vi "Tree.vi"(8 "error in (no error)":errorcluster, 11 "Instrument.Oxford1820":refnum<class "Instrument.OxfordVRM.lvclass">) -> (0 "error out":errorcluster, 3 "Instrument.Oxford1820 out":refnum<class "Instrument.OxfordVRM.lvclass">)   [LabVIEW 2016, in "Instrument.OxfordVRM.lvclass"]
uses:
  Instrument.OxfordVRM.lvclass
  Instrument.Oxford1820 UI/Instrument.OxfordVRM UI.lvclass
  Typedefs/Instrument.Oxford1820.Commands-enum.ctl
  <userlib>/LevyLab/Levylab Instruments/SMOs/Instrument/Instrument.lvclass
  <userlib>/LevyLab/Levylab Instruments/SMOs/RemoteControl/RemoteControl.lvclass
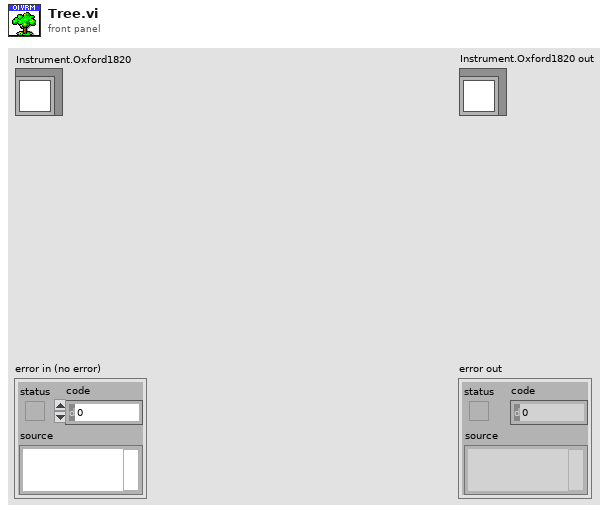
[diagram p1: front panel]
types:
  T1 = typedef "Instrument.OxfordVRM.lvclass/Instrument.Oxford1820.Commands-enum.ctl" = enum16{"setAction", "setTarget", "setSwitchHeat", "setLambda", "setFillMode", "setNeedleValve", "setMagnetField", "getStatus", "getTarget", "getSwitchHeat", "getPSUField", "newcommand", "getMagnetField"}
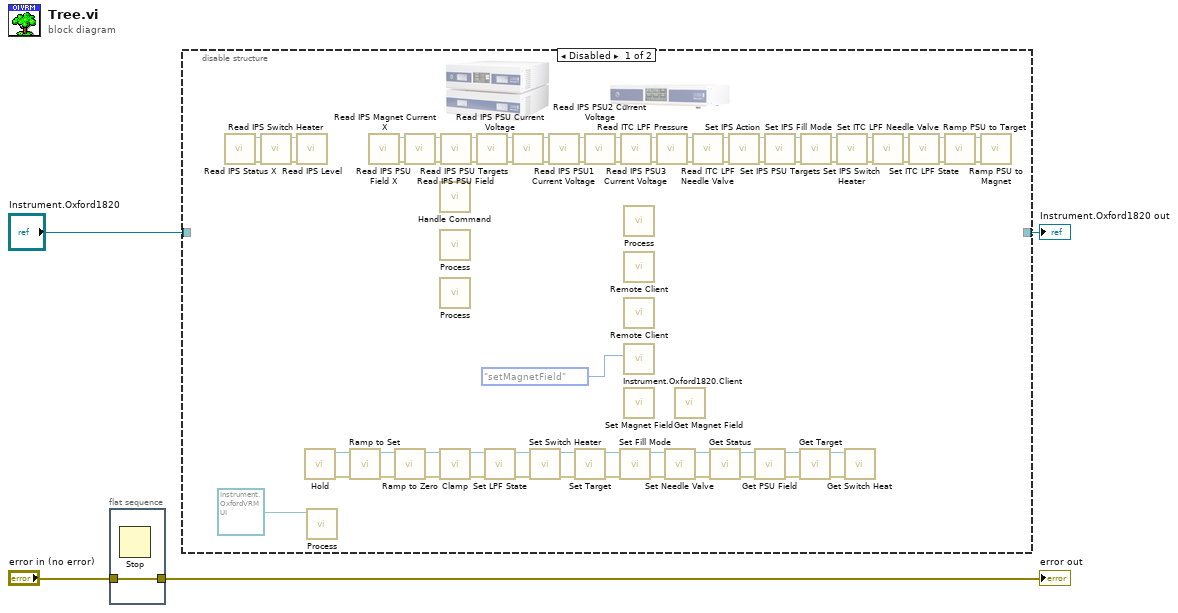
[diagram p0: block diagram]
diagram:
  n1 = flat-sequence {
    tunnel: "error in (no error)" -> [w5]
    tunnel: [w5] -> w4
    frame #0 {
      n2 = Stop() -> ()  [unwired: 1 in]
    }
  }
  n3 = disable-structure shown="Disabled" {
    disable-tunnel: [_ w70] -> w3
    disable-tunnel: "Instrument.Oxford1820" -> [_ w70]
    frame Disabled {
      n4 = call "Read IPS Status X.vi"() -> ("error out"=w67:errorcluster, "Instrument.OxfordVRM out"=w68:refnum<class "Instrument.OxfordVRM.lvclass">)  [unwired: 9 in, 1 out]
      n5 = call "Read IPS Switch Heater.vi"("error in (no error)"=w67, "Instrument.Oxford1820 in"=w68) -> ("error out"=w65:errorcluster, "Instrument.Oxford1820 out"=w66:refnum<class "Instrument.OxfordVRM.lvclass">)  [unwired: 6 in, 2 out]
      n6 = call "Read IPS Level.vi"("error in (no error)"=w65, "Instrument.Oxford1820 in"=w66) -> ()  [unwired: 6 in, 4 out]
      n7 = call "Hold.vi"() -> ("error out"=w33:errorcluster, "Instrument.1820 in"=w34:refnum<class "Instrument.OxfordVRM.lvclass">)  [unwired: 9 in, 1 out]
      n8 = call-dynamic "Process.vi"("Oxford1820 UI in"=refnum<class "Instrument.OxfordVRM UI.lvclass"> refnum ("Instrument.Oxford1820 UI.lvclass")) -> ()  [unwired: 9 in, 2 out]
      n9 = call "Ramp to Set.vi"("error in (no error)"=w33, "Instrument.1820 in"=w34) -> ("error out"=w31:errorcluster, "Instrument.1820 in"=w32:refnum<class "Instrument.OxfordVRM.lvclass">)  [unwired: 7 in, 1 out]
      n10 = call "Read IPS PSU Field X.vi"() -> ("error out"=w63:errorcluster, "Instrument.OxfordVRM out"=w64:refnum<class "Instrument.OxfordVRM.lvclass">)  [unwired: 9 in, 1 out]
      n11 = call "Ramp to Zero.vi"("error in (no error)"=w31, "Instrument.1820 in"=w32) -> ("error out"=w29:errorcluster, "Instrument.1820 in"=w30:refnum<class "Instrument.OxfordVRM.lvclass">)  [unwired: 7 in, 1 out]
      n12 = call "Read IPS Magnet Current X.vi"("error in (no error)"=w63, "Instrument.OxfordVRM in"=w64) -> ("error out"=w61:errorcluster, "Instrument.OxfordVRM out"=w62:refnum<class "Instrument.OxfordVRM.lvclass">)  [unwired: 7 in, 1 out]
      n13 = call-dynamic "Handle Command.vi"() -> ()  [unwired: 8 in, 4 out]
      n14 = call-dynamic "Process.vi"() -> ()  [unwired: 10 in, 2 out]
      n15 = call-dynamic "Process.vi"() -> ()  [unwired: 10 in, 2 out]
      n16 = call "Clamp.vi"("error in (no error)"=w29, "Instrument.1820 in"=w30) -> ("error out"=w27:errorcluster, "Instrument.1820 in"=w28:refnum<class "Instrument.OxfordVRM.lvclass">)  [unwired: 7 in, 1 out]
      n17 = call "Read IPS PSU Field.vi"("error in (no error)"=w61, "Instrument.OxfordVRM in"=w62) -> ("error out"=w59:errorcluster, "Instrument.OxfordVRM out"=w60:refnum<class "Instrument.OxfordVRM.lvclass">)  [unwired: 7 in, 1 out]
      n18 = call "Read IPS PSU Targets.vi"("error in (no error)"=w59, "Instrument.OxfordVRM in"=w60) -> ("error out"=w57:errorcluster, "Instrument.OxfordVRM out"=w58:refnum<class "Instrument.OxfordVRM.lvclass">)  [unwired: 6 in, 2 out]
      n19 = call "Set LPF State.vi"("error in (no error)"=w27, "Instrument.1820 in"=w28) -> ("error out"=w25:errorcluster, "Instrument.1820 in"=w26:refnum<class "Instrument.OxfordVRM.lvclass">)  [unwired: 7 in, 1 out]
      n20 = call "Read IPS PSU Current Voltage.vi"("error in (no error)"=w57, "Instrument.OxfordVRM in"=w58) -> ("error out"=w55:errorcluster, "Instrument.OxfordVRM out"=w56:refnum<class "Instrument.OxfordVRM.lvclass">)  [unwired: 6 in, 2 out]
      n21 = call "Set Switch Heater.vi"("error in (no error)"=w25, "Instrument.1820 in"=w26) -> ("error out"=w23:errorcluster, "Instrument.1820 in"=w24:refnum<class "Instrument.OxfordVRM.lvclass">)  [unwired: 7 in, 1 out]
      n22 = call "Read IPS PSU1 Current Voltage.vi"("error in (no error)"=w55, "Instrument.OxfordVRM in"=w56) -> ("error out"=w53:errorcluster, "Instrument.OxfordVRM out"=w54:refnum<class "Instrument.OxfordVRM.lvclass">)  [unwired: 6 in, 2 out]
      n23 = call "Set Target.vi"("error in (no error)"=w23, "Instrument.1820 in"=w24) -> ("error out"=w21:errorcluster, "Instrument.1820 in"=w22:refnum<class "Instrument.OxfordVRM.lvclass">)  [unwired: 7 in, 1 out]
      n24 = call "Read IPS PSU2 Current Voltage.vi"("error in (no error)"=w53, "Instrument.OxfordVRM in"=w54) -> ("error out"=w51:errorcluster, "Instrument.OxfordVRM out"=w52:refnum<class "Instrument.OxfordVRM.lvclass">)  [unwired: 6 in, 2 out]
      n25 = call "Set Fill Mode.vi"("error in (no error)"=w21, "Instrument.1820 in"=w22) -> ("error out"=w8:errorcluster, "Instrument.1820 in"=w9:refnum<class "Instrument.OxfordVRM.lvclass">)  [unwired: 7 in, 1 out]
      n26 = call "Read IPS PSU3 Current Voltage.vi"("error in (no error)"=w51, "Instrument.OxfordVRM in"=w52) -> ("error out"=w49:errorcluster, "Instrument.OxfordVRM out"=w50:refnum<class "Instrument.OxfordVRM.lvclass">)  [unwired: 6 in, 2 out]
      n27 = call-dynamic "Process.vi"() -> ()  [unwired: 10 in, 2 out]
      n28 = call <userlib>:"Remote Client.vi"() -> ()  [unwired: 8 in, 4 out]
      n29 = call <userlib>:"Remote Client.vi"() -> ()  [unwired: 8 in, 4 out]
      n30 = call "Instrument.Oxford1820.Client.vi"("Commands"=Instrument.Oxford1820.Commands-enum."setMagnetField") -> ()  [unwired: 8 in, 3 out]
      n31 = call-dynamic "Set Magnet Field.vi"() -> ()  [unwired: 10 in, 2 out]
      n32 = call "Read ITC LPF Pressure.vi"("error in (no error)"=w49, "Instrument.Oxford1820 in"=w50) -> ("error out"=w47:errorcluster, "Instrument.Oxford1820 out"=w48:refnum<class "Instrument.OxfordVRM.lvclass">)  [unwired: 7 in, 1 out]
      n33 = call "Set Needle Valve.vi"("error in (no error)"=w8, "Instrument.1820 in"=w9) -> ("error out"=w6:errorcluster, "Instrument.1820 in"=w7:refnum<class "Instrument.OxfordVRM.lvclass">)  [unwired: 7 in, 1 out]
      n34 = call-dynamic "Get Magnet Field.vi"() -> ()  [unwired: 7 in, 5 out]
      n35 = call "Read ITC LPF Needle Valve.vi"("error in (no error)"=w47, "Instrument.Oxford1820 in"=w48) -> ("error out"=w45:errorcluster, "Instrument.Oxford1820 out"=w46:refnum<class "Instrument.OxfordVRM.lvclass">)  [unwired: 7 in, 1 out]
      n36 = call "Get Status.vi"("error in (no error)"=w6, "Instrument.1820 in"=w7) -> ("error out"=w19:errorcluster, "Instrument.1820 in"=w20:refnum<class "Instrument.OxfordVRM.lvclass">)  [unwired: 6 in, 2 out]
      n37 = call "Set IPS Action.vi"("error in (no error)"=w45, "Instrument.OxfordVRM in"=w46) -> ("error out"=w43:errorcluster, "Instrument.OxfordVRM out"=w44:refnum<class "Instrument.OxfordVRM.lvclass">)  [unwired: 7 in, 1 out]
      n38 = call "Get PSU Field.vi"("error in (no error)"=w19, "Instrument.1820 in"=w20) -> ("error out"=w17:errorcluster, "Instrument.1820 in"=w18:refnum<class "Instrument.OxfordVRM.lvclass">)  [unwired: 7 in, 1 out]
      n39 = call "Set IPS PSU Targets.vi"("error in (no error)"=w43, "Instrument.OxfordVRM in"=w44) -> ("error out"=w41:errorcluster, "Instrument.OxfordVRM out"=w42:refnum<class "Instrument.OxfordVRM.lvclass">)  [unwired: 7 in, 1 out]
      n40 = call "Get Target.vi"("error in (no error)"=w17, "Instrument.1820 in"=w18) -> ("error out"=w15:errorcluster, "Instrument.1820 in"=w16:refnum<class "Instrument.OxfordVRM.lvclass">)  [unwired: 6 in, 2 out]
      n41 = call "Set IPS Fill Mode.vi"("error in (no error)"=w41, "Instrument.Oxford1820 in"=w42) -> ("error out"=w39:errorcluster, "Instrument.Oxford1820 out"=w40:refnum<class "Instrument.OxfordVRM.lvclass">)  [unwired: 7 in, 1 out]
      n42 = call "Set IPS Switch Heater.vi"("error in (no error)"=w39, "Instrument.Oxford1820 in"=w40) -> ("error out"=w37:errorcluster, "Instrument.Oxford1820 out"=w38:refnum<class "Instrument.OxfordVRM.lvclass">)  [unwired: 7 in, 1 out]
      n43 = call "Get Switch Heat.vi"("error in (no error)"=w15, "Instrument.1820 in"=w16) -> ()  [unwired: 6 in, 4 out]
      n44 = call "Set ITC LPF Needle Valve.vi"("error in (no error)"=w37, "Instrument.Oxford1820 in"=w38) -> ("error out"=w35:errorcluster, "Instrument.Oxford1820 out"=w36:refnum<class "Instrument.OxfordVRM.lvclass">)  [unwired: 7 in, 1 out]
      n45 = call "Set ITC LPF State.vi"("error in (no error)"=w35, "Instrument.Oxford1820 in"=w36) -> ("error out"=w12:errorcluster, "Instrument.Oxford1820 out"=w13:refnum<class "Instrument.OxfordVRM.lvclass">)  [unwired: 7 in, 1 out]
      n46 = call "Ramp PSU to Target.vi"("error in (no error)"=w12, "Instrument.OxfordVRM in"=w13) -> ("error out"=w10:errorcluster, "Instrument.OxfordVRM out"=w11:refnum<class "Instrument.OxfordVRM.lvclass">)  [unwired: 8 in]
      n47 = call "Ramp PSU to Magnet.vi"("error in (no error)"=w10, "Instrument.VRM in"=w11) -> ()  [unwired: 8 in, 2 out]
    }
    frame Enabled {
    }
  }
  "Instrument.Oxford1820 out" <- w3
  "error out" <- w4
